vi "SimpleMotion.vi"() -> ()   [LabVIEW 2013]
uses:
  Motion/EnableSingle.vi
  Motion/MoveIncSingle.vi
  Motion/WaitSingle.vi
  Motion/DisableSingle.vi
panel:
  out "error out":errorcluster
  out "Position":string
  in  "Distance":dbl=10000.0
  in  "Speed":dbl=5000.0
  in  "Axis Name":string="X"
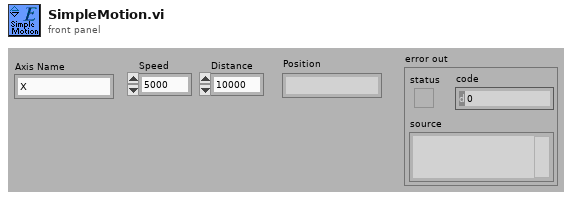
[diagram p1: front panel]
types:
  T1 = typedef "ControllerDiagPacket.ctl" = cluster{"Count":i32, "Packet Time":i64, "Axes":T2[], "error":errorcluster}
  T2 = typedef "AxisDiagPacket.ctl" = cluster{"Axis Name":string, "Acceleration Command":dbl, "Amplifier Temperature":sgl, "Analog Input 0":dbl, "Analog Input 1":dbl, "Analog Output 0":dbl, "Analog Output 1":dbl, "Axis Fault (num)":i32, "Axis Fault (str)":string, "Axis Fault (bits)":cluster{"AmplifierFault":bool, "AmplifierTemperatureFault":bool, "CcwEndOfTravelLimitFault":bool, "CcwSoftwareLimitFault":bool, "CommunicationLostFault":bool, "CwEndOfTravelLimitFault":bool, "CwSoftwareLimitFault":bool, "EmergencyStopFault":bool, "EncoderFault":bool, "ExternalFault":bool, "FeedbackScalingFault":bool, "HallSensorFault":bool, "MarkerSearchFault":bool, "MaxVelocityCommandFault":bool, "MotorTemperatureFault":bool, "None":bool, "OverCurrentFault":bool, "PositionErrorFault":bool, "PositionFeedbackFault":bool, "PowerSupplyFault":bool, "VelocityErrorFault":bool, "VelocityFeedbackFault":bool, "VoltageClampFault":bool}, "Axis Status (num)":i32, "Axis Status (str)":string, "Axis Status (bits)":cluster{"AccelerationPhase":bool, "AutofocusActive":bool, "BrakeOutput":bool, "CalibrationActive":bool, "CalibrationEnabled":bool, "CcwEndOfTravelLimitInput":bool, "CommandShapingFilterDone":bool, "CosineEncoderError":bool, "CurrentClamp":bool, "CwEndOfTravelLimitInput":bool, "DecelerationPhase":bool, "EmergencyStopInput":bool, "Enabled":bool, "GantryMasterActive":bool, "GantryModeActive":bool, "HallAInput":bool, "HallBInput":bool, "HallCInput":bool, "Homed":bool, "HomeLimitInput":bool, "Homing":bool, "InPosition":bool, "InPosition2":bool, "JoystickControl":bool, "MarkerInput":bool, "MasterMotionSuppressed":bool, "MasterSlaveControl":bool, "MotionIsCw":bool, "MoveActive":bool, "None":bool, "PositionCaptureActive":bool, "ServoControl":bool, "SineEncoderError":bool}, "Current Command":sgl, "Current Error":sgl, "Current Feedback":sgl, "Digital Input 0":i32, "Digital Input 1":i32, "Digital Input 2":i32, "Digital Output 0":i32, "Digital Output 1":i32, "Digital Output 2":i32, "Position Feedback Auxiliary":dbl, "Position Command":dbl, "Position Error":dbl, "Position Feedback":dbl, "Program Position Command":dbl, "Program Position Error":dbl, "Program Position Feedback":dbl, "Velocity Command":dbl, "Velocity Error":dbl, "Velocity Feedback":dbl}
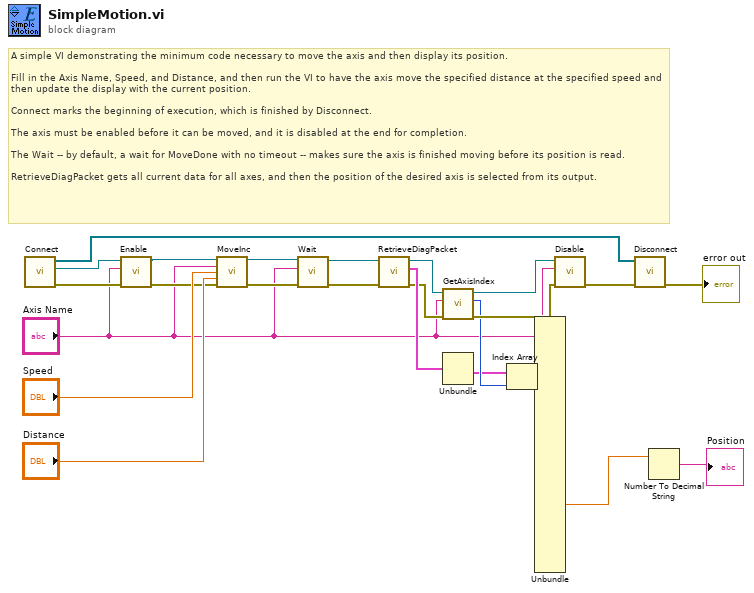
[diagram p0: block diagram]
diagram:
  # "A simple VI demonstrating the minimum code necessary to move the axis and then display its position.\n\nFill in the Axis Name, Speed, and Distance, and then run the VI to have the axis move the specified distance at the specified speed and then update the display with the current position.\n\nConnect marks the beginning of execution, which is finished by Disconnect.\n\nThe axis must be enabled before it can be moved, and it is disabled at the end for completion.\n\nThe Wait -- by default, a wait for MoveDone with no timeout -- makes sure the axis is finished moving before its position is read.\n\nRetrieveDiagPacket gets all current data for all axes, and then the position of the desired axis is selected from its output."
  n1 = call "Connect.vi"() -> ("error out"=w10:errorcluster, "controller"=w11:refnum<k24>, "controllers"=w12:refnum<k24>[])  [unwired: 9 in]
  n2 = call-poly "Enable.vi"("error in (no error)"=w10, "axis name"="Axis Name", "controller in"=w11) -> ("error out"=w9:errorcluster, "controller out"=w8:refnum<k24>)  [unwired: 7 in]
  n3 = call-poly "MoveInc.vi"("controller in"=w8, "axis name"="Axis Name", "speed"="Speed", "distance"="Distance", "error in (no error)"=w9) -> ("controller out"=w3:refnum<k24>, "error out"=w6:errorcluster)  [unwired: 9 in]
  n4 = call-poly "Wait.vi"("error in (no error)"=w6, "axis name"="Axis Name", "controller in"=w3) -> ("error out"=w5:errorcluster, "controller out"=w2:refnum<k24>)  [unwired: 6 in, 1 out]
  n5 = call "RetrieveDiagPacket.vi"("error in (no error)"=w5, "Controller In"=w2) -> ("error out"=w19:errorcluster, "ControllerDiagPacket"=w21:T1, "Controller Out"=w18:refnum<k24>)  [unwired: 7 in]
  n6 = call "GetAxisIndex.vi"("error in (no error)"=w19, "axis name"="Axis Name", "controller in"=w18) -> ("error out"=w16:errorcluster, "axis index"=w15:i32, "controller out"=w17:refnum<k24>)  [unwired: 6 in]
  n7 = Unbundle(w21) -> ("Axes"=w14:T2[])  [unwired: 3 out]
  n8 = Index Array(array=w14, index=w15) -> (element=w13:T2)
  n9 = Unbundle(w13) -> ("Position Command"=w7:dbl)  [unwired: 31 out]
  n10 = call-poly "Disable.vi"("error in (no error)"=w16, "axis name"="Axis Name", "controller in"=w17) -> ("error out"=w24:errorcluster)  [unwired: 7 in, 1 out]
  n11 = call "Disconnect.vi"("error in (no error)"=w24, "controllers"=w12) -> ("error out"=→"error out":errorcluster)  [unwired: 9 in]
  n12 = Number To Decimal String(number=w7) -> (decimal integer string=→"Position":string)  [unwired: 1 in]
